vi "Queue Self Alias.vi"(11 "Hello World Event in":refnum<class "Hello World Event.lvclass">) -> (2 "Queue Self Alias":string)   [LabVIEW 2021, in "Hello World Event.lvlib" / "Hello World Event.lvclass"]
uses:
  Hello World Event.lvclass
  Hello World Event.lvclass/Hello World Event.ctl
  Actor/Event Actor/Event Actor.lvclass
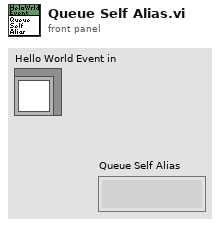
[diagram p1: front panel]
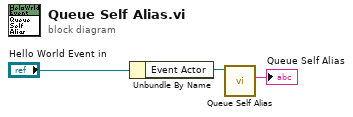
[diagram p0: block diagram]
diagram:
  n1 = Unbundle By Name("Hello World Event in") -> ("Event Actor"=w2:refnum<class "Event Actor.lvclass">)
  n2 = call-dynamic "Queue Self Alias.vi"("Actor in"=w2) -> ("Queue Self Alias"=→"Queue Self Alias":string)  [unwired: 10 in]
